vi "test.vi"() -> ()   [LabVIEW 2016]
uses:
  common_labview_tcpdevice/ts_labview_tcp/tcpTypedefs/TCPSettings.ctl
  IDome/domeTypedefs/azimuth.ctl
  domeCommunicator/ComTypedefs/shortStatus.ctl
  domeCommunicator/ComTypedefs/openingStates.ctl
  IDome/domeTypedefs/openingPercentage.ctl
  domeCommunicator/ComTypedefs/sensorCode.ctl
  domeCommunicator/ComTypedefs/azimimuthPositionStatus.ctl
  IDome/domeTypedefs/direction.ctl
  IDome/domeTypedefs/domeState.ctl
  IDome/domeTypedefs/motionDirection.ctl
  IDome/domeTypedefs/openingMotion.ctl
  domeCommunicator/ComTypedefs/engineeringStatus.ctl
  domeCommunicator/DomeCommunicator.lvclass
  DomeController.lvclass
  domeCommunicator/ComTypedefs/queries.ctl
  domeCommunicator/ComTypedefs/commands.ctl
panel:
  in  "TCP Settings":T1={"IP"="127.0.0.1", "port_low"=50000, "port_up"=50000, "connection_timeout "=1500, "reading_timeout"=1500, "writing_timeout"=1500}
  out "Connected":bool
  in  "disconnect":bool
  in  "connect":bool
  in  "azimuth":T2 min=0.0 max=360.0
  in  "SynchronizedClose":bool
  in  "MoveToAzimuth":bool
  in  "Synchronized Open":bool
  in  "StopAllMotion":bool
  in  "stop":bool
  in  "GetCurrentConfiguration":bool
  in  "SaveCurrentConfiguration":bool
  in  "reverseMotionDelay":dbl
  in  "ReverseMotionDelay":bool
  in  "watchDogTimer":u32
  in  "WatchdogTimer":bool
  in  "enconderCountPer360":dbl
  in  "EncoderCountPer360Deg":bool
  in  "coast":dbl
  in  "Coast":bool
  in  "highSpeedThreshold":dbl
  in  "HighSpeedThreshold":bool
  in  "homePosition":T2 min=0.0 max=360.0
  in  "SetHomePosition":bool
  in  "tolerance":dbl
  in  "Tolerance":bool
  in  "RotateToHomePosition":bool
  in  "CloudSensorOFF":bool
  in  "CloudSensorON":bool
  in  "RainSensorOFF":bool
  in  "CloseMainDoor":bool
  in  "RainSensorON":bool
  in  "AutoShutdownOFF":bool
  in  "AutoShutdownON":bool
  in  "CloseDropoutDoor":bool
  in  "OpenDropoutDoor":bool
  in  "OpenMainDoor":bool
  in  "Status":enum32{"Status", "Advanced Status"}(tab)
  out "shortStatus":T3 {"azimuthAngle" min=0.0 max=360.0; "dropoutDoorOpeningPercentage" min=0.0 max=100.0; "mainDoorOpeningPercentage" min=0.0 max=100.0}
  out "engineeringStatus":T12
  out "Disconnect":errorcluster
  # "Settings"
  # "Main Controls"
  # "degrees"
  # "Advanced Controls"
  # "degrees"
  # "degrees"
  # "degrees"
  # "degrees"
  # "counts"
  # "seconds"
  # "seconds"
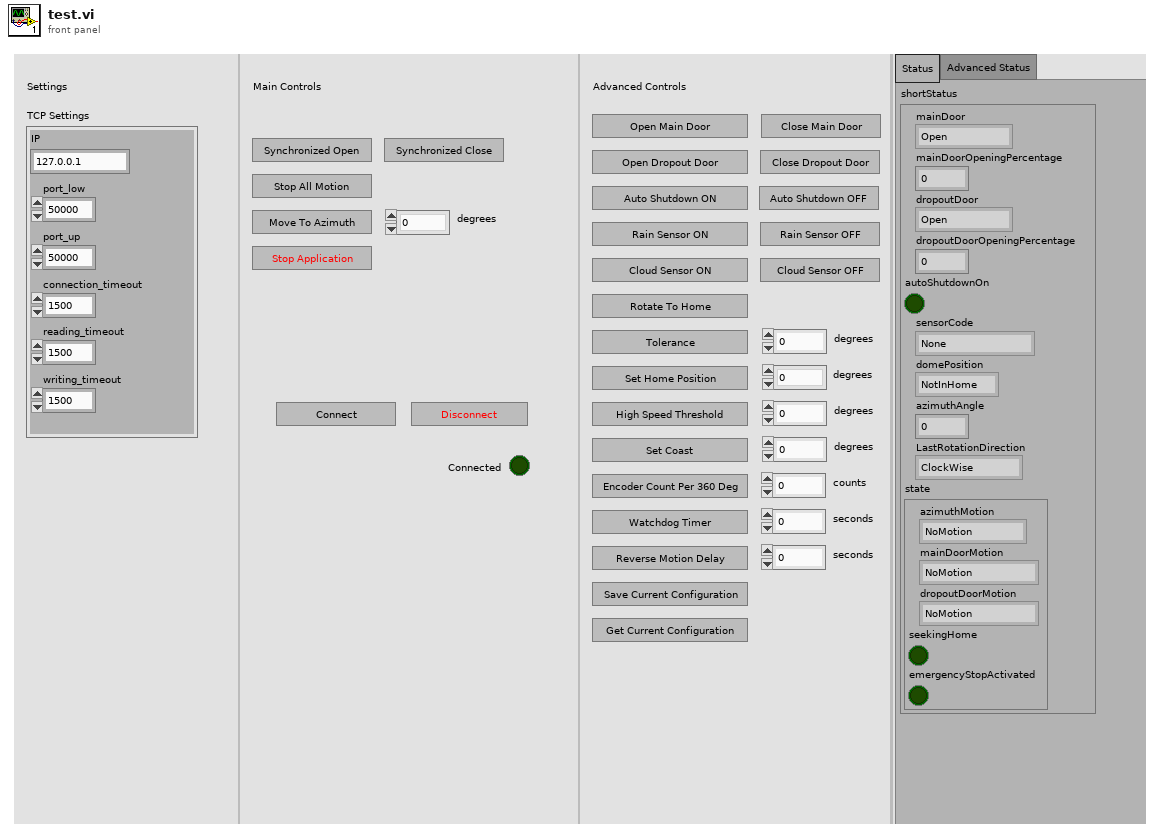
[diagram p1: front panel]
types:
  T1 = typedef "TCPSettings.ctl" = cluster{"IP":string, "port_low":u16, "port_up":u16, "connection_timeout ":i32, "reading_timeout":i32, "writing_timeout":i32}
  T2 = typedef "azimuth.ctl" = dbl
  T3 = typedef "shortStatus.ctl" = cluster{"mainDoor":T4, "mainDoorOpeningPercentage":T5, "dropoutDoor":T4, "dropoutDoorOpeningPercentage":T5, "autoShutdownOn":bool, "sensorCode":T6, "domePosition":T7, "azimuthAngle":T2, "LastRotationDirection":T8, "state":T9}
  T4 = typedef "openingStates.ctl" = enum16{"Open", "Shut", "Ajar"}
  T5 = typedef "openingPercentage.ctl" = dbl
  T6 = typedef "sensorCode.ctl" = enum16{"None", "RainSnowSensorTriggered", "CloudSensorTriggered", "BothSensorsTriggered"}
  T7 = typedef "azimimuthPositionStatus.ctl" = enum16{"NotInHome", "Home"}
  T8 = typedef "direction.ctl" = enum16{"ClockWise", "CounterClockWise"}
  T9 = typedef "domeState.ctl" = cluster{"azimuthMotion":T10, "mainDoorMotion":T11, "dropoutDoorMotion ":T11, "seekingHome":bool, "emergencyStopActivated":bool}
  T10 = typedef "motionDirection.ctl" = enum16{"NoMotion", "MovingClockWise", "MovingCounterClockWise"}
  T11 = typedef "openingMotion.ctl" = enum16{"NoMotion", "Opening", "Closing"}
  T12 = typedef "engineeringStatus.ctl" = cluster{"SCBRatioLinkOK":bool, "homeAzimuth":dbl, "highSpeed":dbl, "coast":dbl, "tolerance":dbl, "enconderCountPer360":u32, "encoderCount":u32, "lastAzimuthGoTo":dbl, "rainSnowSensoEnabled":bool, "cloudSensorEnabled":bool, "watchdogResetTime":dbl, "dropoutTimer":dbl, "reverseDelay":dbl, "mainDoorEncoderClosed":u32, "mainDoorEncoderOpened":u32, "dropoutEncoderClosed":u32, "dropoutEncoderOpened":u32}
  T13 = typedef "queries.ctl" = enum16{"ShortStatus", "FullEngineeringStatus", "RecallLastSavedConfiguration"}
  T14 = typedef "commands.ctl" = enum16{"StopAllMotion", "CloseMainDoor", "OpenMainDoor", "CloseDropoutDoor", "OpenDropoutDoor", "SynchronizedOpen", "SynchronizedClose", "AutoShutDownOn", "AutoShutDownOff", "RainOn", "RainOff", "CloudSensorOn", "CloudSensorOff", "RotateToHomePosition", "MoveToAzimuth", "SetTolerance", "DefineHomePosition", "HighSpeedThreshold", "SetCoast", "SetEncoderCountFor360", "SetWatchDogTimer", "SetReverseDirectionMotionDelay", "SaveCurrentConfiguration"}
  T15 = typedef "fullEngineeringStatus.ctl" = cluster{"shortStatus":T3, "engineeringStatus":T12}
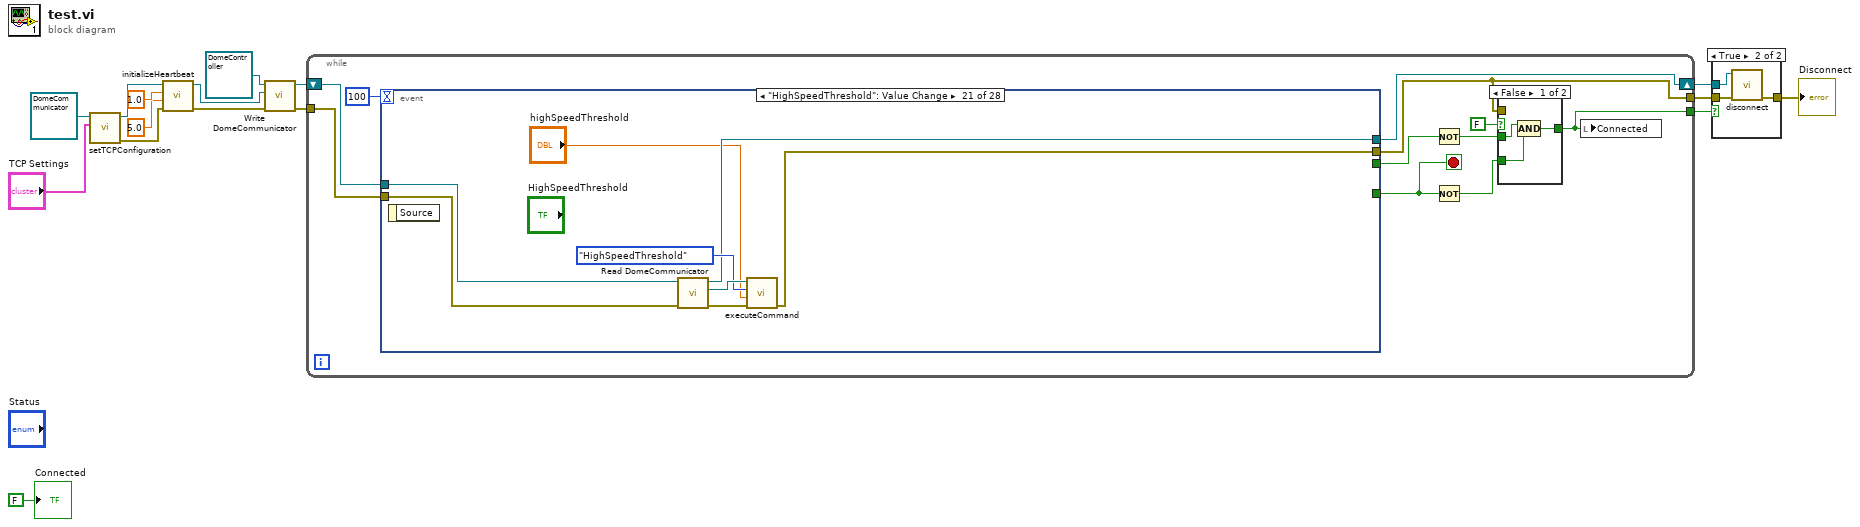
[diagram p0: block diagram]
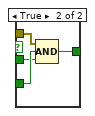
[diagram p3: hidden frame]
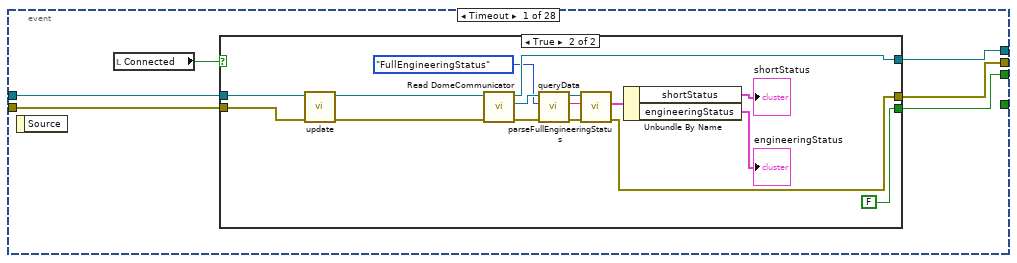
[diagram p4: hidden frame]
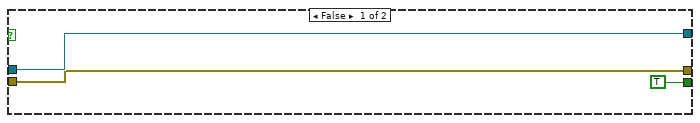
[diagram p5: hidden frame]
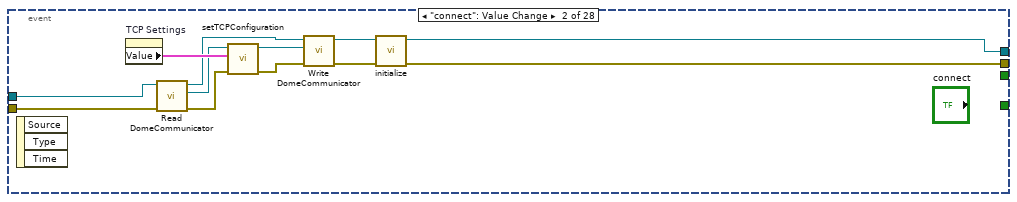
[diagram p6: hidden frame]
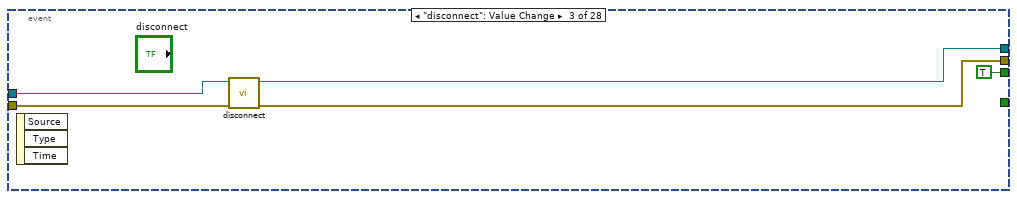
[diagram p7: hidden frame]
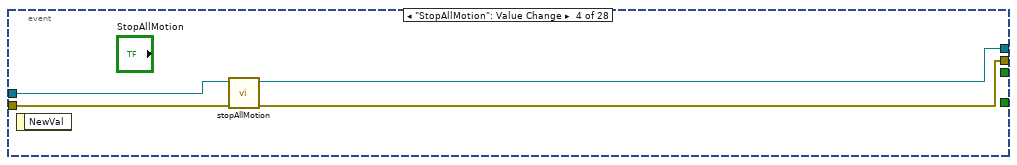
[diagram p8: hidden frame]
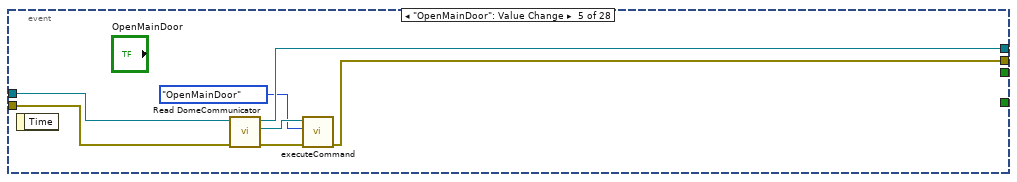
[diagram p9: hidden frame]
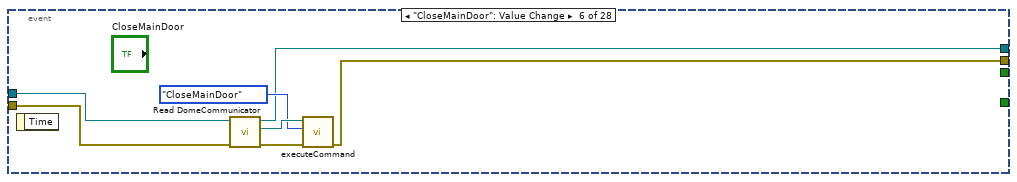
[diagram p10: hidden frame]
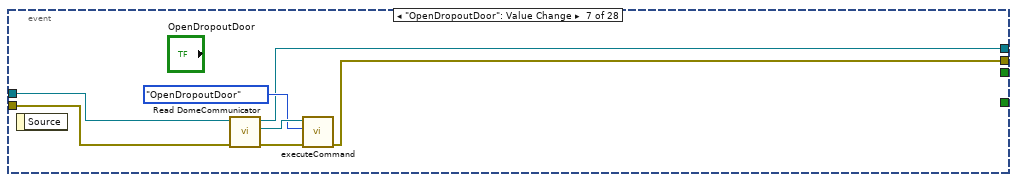
[diagram p11: hidden frame]
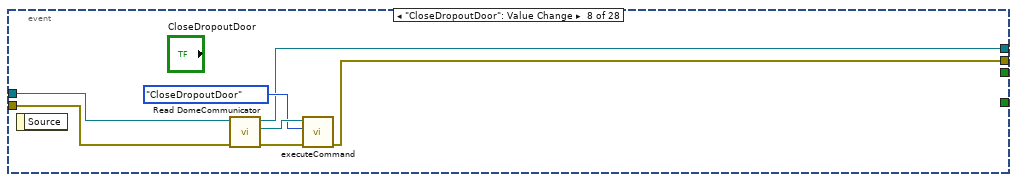
[diagram p12: hidden frame]
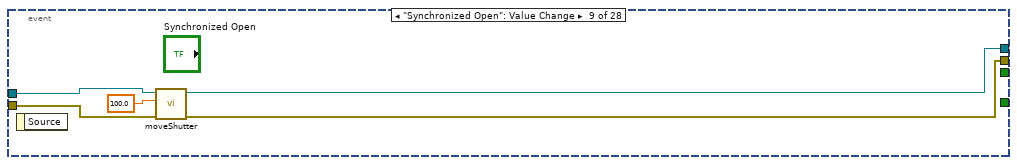
[diagram p13: hidden frame]
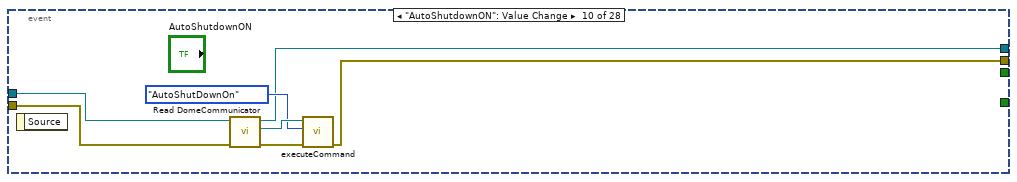
[diagram p14: hidden frame]
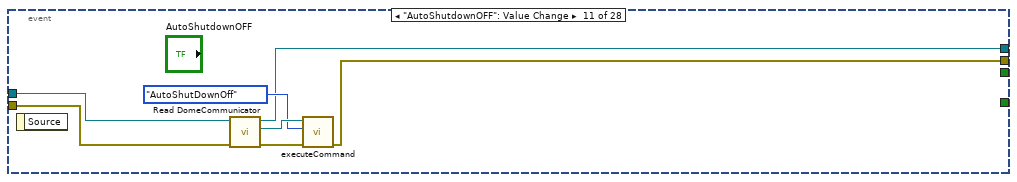
[diagram p15: hidden frame]
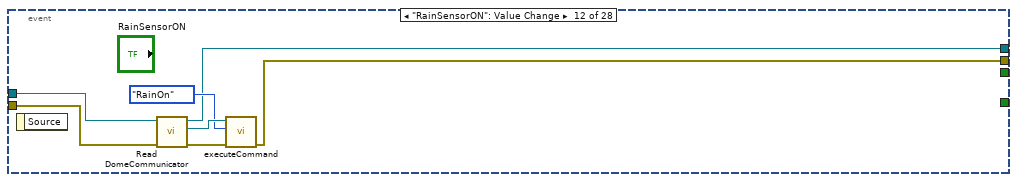
[diagram p16: hidden frame]
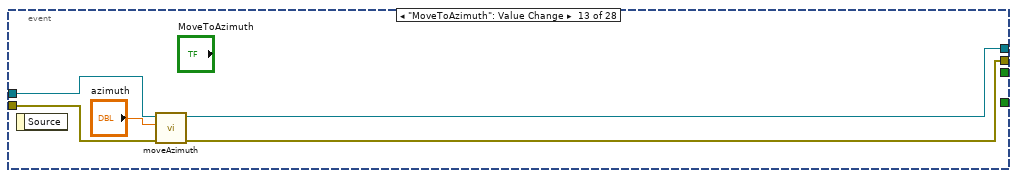
[diagram p17: hidden frame]
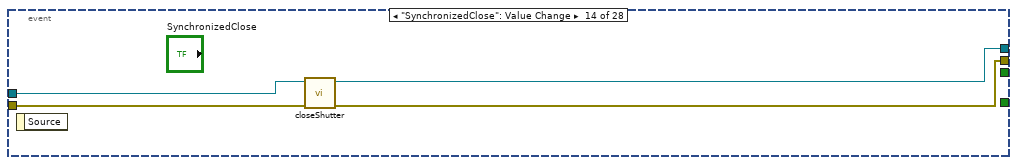
[diagram p18: hidden frame]
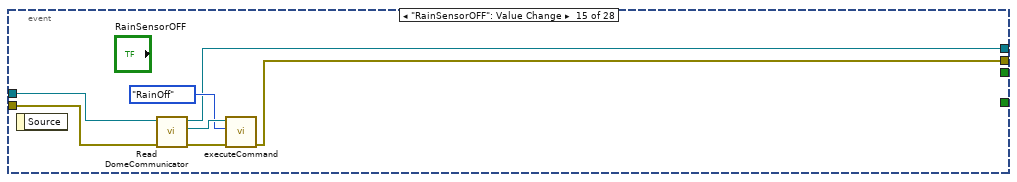
[diagram p19: hidden frame]
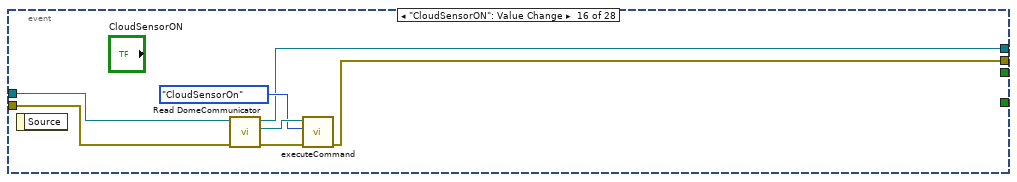
[diagram p20: hidden frame]
diagram:
  n1 = call-dynamic "setTCPConfiguration.vi"("Settings"="TCP Settings", "tcpDevice in"=refnum<class "DomeCommunicator.lvclass"> refnum ("domeCommunicator.lvclass")) -> ("error out"=w5:errorcluster, "tcpDevice out"=w6:refnum<class "DomeCommunicator.lvclass">)  [unwired: 8 in]
  n2 = call-dynamic "initializeHeartbeat.vi"("error in (no error)"=w5, "timeout"=5.0, "period"=1.0, "tcpDevice in"=w6) -> ("error out"=w10:errorcluster, "tcpDevice out"=w9:refnum<class "DomeCommunicator.lvclass">)  [unwired: 6 in]
  n3 = call-dynamic "Write DomeCommunicator.vi"("error in (no error)"=w10, "DomeCommunicator.lvclass"=w9, "DomeController in"=refnum<class "DomeController.lvclass"> refnum) -> ("error out"=w3:errorcluster, "DomeController out"=w4:refnum<class "DomeController.lvclass">)  [unwired: 7 in]
  n4 = while {
    tunnel: w3 -> [w25]
    tunnel: [w18] -> w12
    shift-right: [w26] -> w7
    shift-left: w4 -> [w24]
    tunnel: [w19] -> w2
    stop <- w23 stop-if-true
    n5 = event shown="[20] \"HighSpeedThreshold\": Value Change" {
      selector: _ -> [_ _ _ _ _ _ _ _ _ _ _ _ _ _ _ _ _ _ _ _ _ _ _ _ _ _ _ _]
      dyn-events: _ -> [_ _ _ _ _ _ _ _ _ _ _ _ _ _ _ _ _ _ _ _ _ _ _ _ _ _ _ _]
      timeout: 100 -> [_ _ _ _ _ _ _ _ _ _ _ _ _ _ _ _ _ _ _ _ _ _ _ _ _ _ _ _]
      tunnel: w25 -> [w39 w63 w75 w79 w86 w91 w97 w104 w112 w116 w123 w130 w137 w142 w146 w153 w160 w167 w176 w183 w191 w199 w207 w215 w223 w230 w242 w243]
      tunnel: w24 -> [w40 w64 w76 w80 w87 w90 w98 w105 w113 w117 w124 w131 w139 w143 w147 w154 w161 w168 w175 w184 w192 w200 w208 w216 w224 w231 w241 w244]
      tunnel: [w38 w70 w73 w77 w82 w89 w95 w102 w110 w114 w121 w128 w138 w140 w144 w151 w158 w165 w174 w181 w189 w197 w205 w213 w221 w228 w240 w244] -> w26
      tunnel: [w37 w71 w74 w78 w83 w88 w96 w103 w111 w115 w122 w129 w135 w141 w145 w152 w159 w166 w173 w182 w190 w198 w206 w214 w222 w229 w236 w243] -> w18
      tunnel: [_ _ _ _ _ _ _ _ _ _ _ _ _ _ _ _ _ _ _ _ _ _ _ _ _ _ _ "stop"] -> w23
      tunnel: [w35 _ TRUE ("stop") _ _ _ _ _ _ _ _ _ _ _ _ _ _ _ _ _ _ _ _ _ _ _ _ _] -> w21
      event Timeout {
        n6 = event-data() -> ()  [unwired: 1 in, 1 out]
        n7 = local read "Connected"() -> (w36:bool)
        n8 = case shown="True" w36 {
          tunnel: w40 -> [w43 w59]
          tunnel: w39 -> [w42 w58]
          tunnel: [w43 w55] -> w38
          tunnel: [w42 w50] -> w37
          tunnel: [TRUE ("stop") FALSE ("stop")] -> w35
          frame False {
          }
          frame True {
            n9 = call-dynamic "update.vi"("error in (no error)"=w58, "DomeController in"=w59) -> ("error out"=w56:errorcluster, "DomeController out"=w57:refnum<class "DomeController.lvclass">)  [unwired: 8 in]
            n10 = call-dynamic "Read DomeCommunicator.vi"("error in (no error)"=w56, "DomeController in"=w57) -> ("error out"=w53:errorcluster, "DomeCommunicator.lvclass"=w54:refnum<class "DomeCommunicator.lvclass">, "DomeController out"=w55:refnum<class "DomeController.lvclass">)  [unwired: 7 in]
            n11 = call "queryData.vi"("error in (no error)"=w53, "queries"=queries."FullEngineeringStatus", "DomeCommunicator in"=w54) -> ("error out"=w51:errorcluster, "response"=w48:string, "DomeCommunicator out"=w49:refnum<class "DomeCommunicator.lvclass">)  [unwired: 5 in, 1 out]
            n12 = call "parseFullEngineeringStatus.vi"("error in (no error)"=w51, "engineeringStatusString"=w48, "DomeCommunicator in"=w49) -> ("error out"=w50:errorcluster, "fullEngineeringStatus"=w47:T15)  [unwired: 6 in, 1 out]
            n13 = Unbundle By Name(w47) -> ("shortStatus"=→"shortStatus":T3, "engineeringStatus"=→"engineeringStatus":T12)
          }
        }
      }
      event "connect": Value Change {
        n14 = event-data() -> ()  [unwired: 1 in, 3 out]
        n15 = property on="TCP Settings" class="Clust (strict)"() -> ("Value"=w65:T1)  [unwired: 2 in, 2 out]
        n16 = call-dynamic "Read DomeCommunicator.vi"("error in (no error)"=w63, "DomeController in"=w64) -> ("error out"=w60:errorcluster, "DomeCommunicator.lvclass"=w62:refnum<class "DomeCommunicator.lvclass">, "DomeController out"=w61:refnum<class "DomeController.lvclass">)  [unwired: 7 in]
        n17 = call-dynamic "setTCPConfiguration.vi"("error in (no error)"=w60, "Settings"=w65, "tcpDevice in"=w62) -> ("error out"=w69:errorcluster, "tcpDevice out"=w66:refnum<class "DomeCommunicator.lvclass">)  [unwired: 7 in]
        n18 = call-dynamic "Write DomeCommunicator.vi"("error in (no error)"=w69, "DomeCommunicator.lvclass"=w66, "DomeController in"=w61) -> ("error out"=w68:errorcluster, "DomeController out"=w67:refnum<class "DomeController.lvclass">)  [unwired: 7 in]
        n19 = call-dynamic "initialize.vi"("error in (no error)"=w68, "DomeController in"=w67) -> ("error out"=w71:errorcluster, "DomeController out"=w70:refnum<class "DomeController.lvclass">)  [unwired: 8 in]
      }
      event "disconnect": Value Change {
        n20 = event-data() -> ()  [unwired: 1 in, 3 out]
        n21 = call-dynamic "disconnect.vi"("error in (no error)"=w75, "DomeController in"=w76) -> ("error out"=w74:errorcluster, "DomeController out"=w73:refnum<class "DomeController.lvclass">)  [unwired: 8 in]
      }
      event "StopAllMotion": Value Change {
        n22 = event-data() -> ()  [unwired: 1 in, 1 out]
        n23 = call-dynamic "stopAllMotion.vi"("error in (no error)"=w79, "DomeController in"=w80) -> ("error out"=w78:errorcluster, "DomeController out"=w77:refnum<class "DomeController.lvclass">)  [unwired: 8 in]
      }
      event "OpenMainDoor": Value Change {
        n24 = event-data() -> ()  [unwired: 1 in, 1 out]
        n25 = call-dynamic "Read DomeCommunicator.vi"("error in (no error)"=w86, "DomeController in"=w87) -> ("error out"=w84:errorcluster, "DomeCommunicator.lvclass"=w85:refnum<class "DomeCommunicator.lvclass">, "DomeController out"=w82:refnum<class "DomeController.lvclass">)  [unwired: 7 in]
        n26 = call "executeCommand.vi"("error in (no error)"=w84, "Command"=commands."OpenMainDoor", "DomeCommunicator in"=w85) -> ("error out"=w83:errorcluster)  [unwired: 7 in, 1 out]
      }
      event "CloseMainDoor": Value Change {
        n27 = event-data() -> ()  [unwired: 1 in, 1 out]
        n28 = call-dynamic "Read DomeCommunicator.vi"("error in (no error)"=w91, "DomeController in"=w90) -> ("error out"=w93:errorcluster, "DomeCommunicator.lvclass"=w94:refnum<class "DomeCommunicator.lvclass">, "DomeController out"=w89:refnum<class "DomeController.lvclass">)  [unwired: 7 in]
        n29 = call "executeCommand.vi"("error in (no error)"=w93, "Command"=commands."CloseMainDoor", "DomeCommunicator in"=w94) -> ("error out"=w88:errorcluster)  [unwired: 7 in, 1 out]
      }
      event "OpenDropoutDoor": Value Change {
        n30 = event-data() -> ()  [unwired: 1 in, 1 out]
        n31 = call-dynamic "Read DomeCommunicator.vi"("error in (no error)"=w97, "DomeController in"=w98) -> ("error out"=w100:errorcluster, "DomeCommunicator.lvclass"=w101:refnum<class "DomeCommunicator.lvclass">, "DomeController out"=w95:refnum<class "DomeController.lvclass">)  [unwired: 7 in]
        n32 = call "executeCommand.vi"("error in (no error)"=w100, "Command"=commands."OpenDropoutDoor", "DomeCommunicator in"=w101) -> ("error out"=w96:errorcluster)  [unwired: 7 in, 1 out]
      }
      event "CloseDropoutDoor": Value Change {
        n33 = event-data() -> ()  [unwired: 1 in, 1 out]
        n34 = call-dynamic "Read DomeCommunicator.vi"("error in (no error)"=w104, "DomeController in"=w105) -> ("error out"=w107:errorcluster, "DomeCommunicator.lvclass"=w108:refnum<class "DomeCommunicator.lvclass">, "DomeController out"=w102:refnum<class "DomeController.lvclass">)  [unwired: 7 in]
        n35 = call "executeCommand.vi"("error in (no error)"=w107, "Command"=commands."CloseDropoutDoor", "DomeCommunicator in"=w108) -> ("error out"=w103:errorcluster)  [unwired: 7 in, 1 out]
      }
      event "Synchronized Open": Value Change {
        n36 = event-data() -> ()  [unwired: 1 in, 1 out]
        n37 = call-dynamic "moveShutter.vi"("error in (no error)"=w112, "openingPercentage"=T5 100.0, "DomeController in"=w113) -> ("error out"=w111:errorcluster, "DomeController out"=w110:refnum<class "DomeController.lvclass">)  [unwired: 7 in]
      }
      event "AutoShutdownON": Value Change {
        n38 = event-data() -> ()  [unwired: 1 in, 1 out]
        n39 = call-dynamic "Read DomeCommunicator.vi"("error in (no error)"=w116, "DomeController in"=w117) -> ("error out"=w119:errorcluster, "DomeCommunicator.lvclass"=w120:refnum<class "DomeCommunicator.lvclass">, "DomeController out"=w114:refnum<class "DomeController.lvclass">)  [unwired: 7 in]
        n40 = call "executeCommand.vi"("error in (no error)"=w119, "Command"=commands."AutoShutDownOn", "DomeCommunicator in"=w120) -> ("error out"=w115:errorcluster)  [unwired: 7 in, 1 out]
      }
      event "AutoShutdownOFF": Value Change {
        n41 = event-data() -> ()  [unwired: 1 in, 1 out]
        n42 = call-dynamic "Read DomeCommunicator.vi"("error in (no error)"=w123, "DomeController in"=w124) -> ("error out"=w126:errorcluster, "DomeCommunicator.lvclass"=w127:refnum<class "DomeCommunicator.lvclass">, "DomeController out"=w121:refnum<class "DomeController.lvclass">)  [unwired: 7 in]
        n43 = call "executeCommand.vi"("error in (no error)"=w126, "Command"=commands."AutoShutDownOff", "DomeCommunicator in"=w127) -> ("error out"=w122:errorcluster)  [unwired: 7 in, 1 out]
      }
      event "RainSensorON": Value Change {
        n44 = event-data() -> ()  [unwired: 1 in, 1 out]
        n45 = call-dynamic "Read DomeCommunicator.vi"("error in (no error)"=w130, "DomeController in"=w131) -> ("error out"=w133:errorcluster, "DomeCommunicator.lvclass"=w134:refnum<class "DomeCommunicator.lvclass">, "DomeController out"=w128:refnum<class "DomeController.lvclass">)  [unwired: 7 in]
        n46 = call "executeCommand.vi"("error in (no error)"=w133, "Command"=commands."RainOn", "DomeCommunicator in"=w134) -> ("error out"=w129:errorcluster)  [unwired: 7 in, 1 out]
      }
      event "MoveToAzimuth": Value Change {
        n47 = event-data() -> ()  [unwired: 1 in, 1 out]
        n48 = call-dynamic "moveAzimuth.vi"("error in (no error)"=w137, "azimuth"="azimuth", "DomeController in"=w139) -> ("error out"=w135:errorcluster, "DomeController out"=w138:refnum<class "DomeController.lvclass">)  [unwired: 7 in]
      }
      event "SynchronizedClose": Value Change {
        n49 = event-data() -> ()  [unwired: 1 in, 1 out]
        n50 = call-dynamic "closeShutter.vi"("error in (no error)"=w142, "DomeController in"=w143) -> ("error out"=w141:errorcluster, "DomeController out"=w140:refnum<class "DomeController.lvclass">)  [unwired: 8 in]
      }
      event "RainSensorOFF": Value Change {
        n51 = event-data() -> ()  [unwired: 1 in, 1 out]
        n52 = call-dynamic "Read DomeCommunicator.vi"("error in (no error)"=w146, "DomeController in"=w147) -> ("error out"=w149:errorcluster, "DomeCommunicator.lvclass"=w150:refnum<class "DomeCommunicator.lvclass">, "DomeController out"=w144:refnum<class "DomeController.lvclass">)  [unwired: 7 in]
        n53 = call "executeCommand.vi"("error in (no error)"=w149, "Command"=commands."RainOff", "DomeCommunicator in"=w150) -> ("error out"=w145:errorcluster)  [unwired: 7 in, 1 out]
      }
      event "CloudSensorON": Value Change {
        n54 = event-data() -> ()  [unwired: 1 in, 1 out]
        n55 = call-dynamic "Read DomeCommunicator.vi"("error in (no error)"=w153, "DomeController in"=w154) -> ("error out"=w156:errorcluster, "DomeCommunicator.lvclass"=w157:refnum<class "DomeCommunicator.lvclass">, "DomeController out"=w151:refnum<class "DomeController.lvclass">)  [unwired: 7 in]
        n56 = call "executeCommand.vi"("error in (no error)"=w156, "Command"=commands."CloudSensorOn", "DomeCommunicator in"=w157) -> ("error out"=w152:errorcluster)  [unwired: 7 in, 1 out]
      }
      event "CloudSensorOFF": Value Change {
        n57 = event-data() -> ()  [unwired: 1 in, 1 out]
        n58 = call-dynamic "Read DomeCommunicator.vi"("error in (no error)"=w160, "DomeController in"=w161) -> ("error out"=w163:errorcluster, "DomeCommunicator.lvclass"=w164:refnum<class "DomeCommunicator.lvclass">, "DomeController out"=w158:refnum<class "DomeController.lvclass">)  [unwired: 7 in]
        n59 = call "executeCommand.vi"("error in (no error)"=w163, "Command"=commands."CloudSensorOff", "DomeCommunicator in"=w164) -> ("error out"=w159:errorcluster)  [unwired: 7 in, 1 out]
      }
      event "RotateToHomePosition": Value Change {
        n60 = event-data() -> ()  [unwired: 1 in, 1 out]
        n61 = call-dynamic "Read DomeCommunicator.vi"("error in (no error)"=w167, "DomeController in"=w168) -> ("error out"=w170:errorcluster, "DomeCommunicator.lvclass"=w171:refnum<class "DomeCommunicator.lvclass">, "DomeController out"=w165:refnum<class "DomeController.lvclass">)  [unwired: 7 in]
        n62 = call "executeCommand.vi"("error in (no error)"=w170, "Command"=commands."RotateToHomePosition", "DomeCommunicator in"=w171) -> ("error out"=w166:errorcluster)  [unwired: 7 in, 1 out]
      }
      event "Tolerance": Value Change {
        n63 = event-data() -> ()  [unwired: 1 in, 1 out]
        n64 = call-dynamic "Read DomeCommunicator.vi"("error in (no error)"=w176, "DomeController in"=w175) -> ("error out"=w178:errorcluster, "DomeCommunicator.lvclass"=w179:refnum<class "DomeCommunicator.lvclass">, "DomeController out"=w174:refnum<class "DomeController.lvclass">)  [unwired: 7 in]
        n65 = call "executeCommand.vi"("error in (no error)"=w178, "Variant"="tolerance", "Command"=commands."SetTolerance", "DomeCommunicator in"=w179) -> ("error out"=w173:errorcluster)  [unwired: 6 in, 1 out]
      }
      event "SetHomePosition": Value Change {
        n66 = event-data() -> ()  [unwired: 1 in, 1 out]
        n67 = call-dynamic "Read DomeCommunicator.vi"("error in (no error)"=w183, "DomeController in"=w184) -> ("error out"=w186:errorcluster, "DomeCommunicator.lvclass"=w187:refnum<class "DomeCommunicator.lvclass">, "DomeController out"=w181:refnum<class "DomeController.lvclass">)  [unwired: 7 in]
        n68 = call "executeCommand.vi"("error in (no error)"=w186, "Variant"="homePosition", "Command"=commands."DefineHomePosition", "DomeCommunicator in"=w187) -> ("error out"=w182:errorcluster)  [unwired: 6 in, 1 out]
      }
      event "HighSpeedThreshold": Value Change {
        n69 = event-data() -> ()  [unwired: 1 in, 1 out]
        n70 = call-dynamic "Read DomeCommunicator.vi"("error in (no error)"=w191, "DomeController in"=w192) -> ("error out"=w194:errorcluster, "DomeCommunicator.lvclass"=w195:refnum<class "DomeCommunicator.lvclass">, "DomeController out"=w189:refnum<class "DomeController.lvclass">)  [unwired: 7 in]
        n71 = call "executeCommand.vi"("error in (no error)"=w194, "Variant"="highSpeedThreshold", "Command"=commands."HighSpeedThreshold", "DomeCommunicator in"=w195) -> ("error out"=w190:errorcluster)  [unwired: 6 in, 1 out]
      }
      event "Coast": Value Change {
        n72 = event-data() -> ()  [unwired: 1 in, 1 out]
        n73 = call-dynamic "Read DomeCommunicator.vi"("error in (no error)"=w199, "DomeController in"=w200) -> ("error out"=w202:errorcluster, "DomeCommunicator.lvclass"=w203:refnum<class "DomeCommunicator.lvclass">, "DomeController out"=w197:refnum<class "DomeController.lvclass">)  [unwired: 7 in]
        n74 = call "executeCommand.vi"("error in (no error)"=w202, "Variant"="coast", "Command"=commands."SetCoast", "DomeCommunicator in"=w203) -> ("error out"=w198:errorcluster)  [unwired: 6 in, 1 out]
      }
      event "EncoderCountPer360Deg": Value Change {
        n75 = event-data() -> ()  [unwired: 1 in, 1 out]
        n76 = call-dynamic "Read DomeCommunicator.vi"("error in (no error)"=w207, "DomeController in"=w208) -> ("error out"=w210:errorcluster, "DomeCommunicator.lvclass"=w211:refnum<class "DomeCommunicator.lvclass">, "DomeController out"=w205:refnum<class "DomeController.lvclass">)  [unwired: 7 in]
        n77 = call "executeCommand.vi"("error in (no error)"=w210, "Variant"="enconderCountPer360", "Command"=commands."SetEncoderCountFor360", "DomeCommunicator in"=w211) -> ("error out"=w206:errorcluster)  [unwired: 6 in, 1 out]
      }
      event "WatchdogTimer": Value Change {
        n78 = event-data() -> ()  [unwired: 1 in, 1 out]
        n79 = call-dynamic "Read DomeCommunicator.vi"("error in (no error)"=w215, "DomeController in"=w216) -> ("error out"=w218:errorcluster, "DomeCommunicator.lvclass"=w219:refnum<class "DomeCommunicator.lvclass">, "DomeController out"=w213:refnum<class "DomeController.lvclass">)  [unwired: 7 in]
        n80 = call "executeCommand.vi"("error in (no error)"=w218, "Variant"="watchDogTimer", "Command"=commands."SetWatchDogTimer", "DomeCommunicator in"=w219) -> ("error out"=w214:errorcluster)  [unwired: 6 in, 1 out]
      }
      event "ReverseMotionDelay": Value Change {
        n81 = event-data() -> ()  [unwired: 1 in, 1 out]
        n82 = call-dynamic "Read DomeCommunicator.vi"("error in (no error)"=w223, "DomeController in"=w224) -> ("error out"=w226:errorcluster, "DomeCommunicator.lvclass"=w227:refnum<class "DomeCommunicator.lvclass">, "DomeController out"=w221:refnum<class "DomeController.lvclass">)  [unwired: 7 in]
        n83 = call "executeCommand.vi"("error in (no error)"=w226, "Variant"="reverseMotionDelay", "Command"=commands."SetReverseDirectionMotionDelay", "DomeCommunicator in"=w227) -> ("error out"=w222:errorcluster)  [unwired: 6 in, 1 out]
      }
      event "SaveCurrentConfiguration": Value Change {
        n84 = event-data() -> ()  [unwired: 1 in, 1 out]
        n85 = call-dynamic "Read DomeCommunicator.vi"("error in (no error)"=w230, "DomeController in"=w231) -> ("error out"=w233:errorcluster, "DomeCommunicator.lvclass"=w234:refnum<class "DomeCommunicator.lvclass">, "DomeController out"=w228:refnum<class "DomeController.lvclass">)  [unwired: 7 in]
        n86 = call "executeCommand.vi"("error in (no error)"=w233, "Command"=commands."SaveCurrentConfiguration", "DomeCommunicator in"=w234) -> ("error out"=w229:errorcluster)  [unwired: 7 in, 1 out]
      }
      event "GetCurrentConfiguration": Value Change {
        n87 = event-data() -> ()  [unwired: 1 in, 1 out]
        n88 = call-dynamic "Read DomeCommunicator.vi"("error in (no error)"=w242, "DomeController in"=w241) -> ("error out"=w238:errorcluster, "DomeCommunicator.lvclass"=w239:refnum<class "DomeCommunicator.lvclass">, "DomeController out"=w240:refnum<class "DomeController.lvclass">)  [unwired: 7 in]
        n89 = call "queryData.vi"("error in (no error)"=w238, "queries"=queries."RecallLastSavedConfiguration", "DomeCommunicator in"=w239) -> ("error out"=w236:errorcluster, "response"=w235:string)  [unwired: 5 in, 2 out]
        n90 = call "Display Message to User"("Message"=w235) -> ()  [unwired: 9 in, 2 out]
      }
      event "stop": Value Change {
        n91 = event-data() -> ()  [unwired: 1 in, 1 out]
      }
    }
    n92 = Not(x=w21) -> (.not. x?=w20:bool)
    n93 = Not(x=w23) -> (.not. x?=w22:bool)
    n94 = case shown="False" FALSE {
      tunnel: w22 -> [w28 w34]
      tunnel: w20 -> [w29 w33]
      tunnel: [w30 w32] -> w19
      tunnel: w18 -> [_ w31]
      frame False {
        n95 = Compound Arithmetic op=AND(w29, w28) -> (w30:bool)
      }
      frame True {
        n96 = Compound Arithmetic op=AND(w31, w34, w33) -> (w32:bool)
      }
    }
    n97 = local write "Connected"(w19) -> ()
  }
  n98 = case shown="True" w2 {
    tunnel: w12 -> [w246 w249]
    tunnel: [w246 w248] -> w11
    tunnel: w7 -> [_ w247]
    frame False {
    }
    frame True {
      n99 = call-dynamic "disconnect.vi"("error in (no error)"=w249, "DomeController in"=w247) -> ("error out"=w248:errorcluster)  [unwired: 8 in, 1 out]
    }
  }
  "Disconnect" <- w11
  "Connected" <- FALSE ("Connected")
